vi "Save Excel Reports.vi"(11 "NI_report in":refnum<class "NI_report.lvclass">) -> ()   [LabVIEW 2019]
uses:
  <vilib>/Utility/NIReport.llb/NI_report.lvclass
  Global Tektronix Report Cells.vi
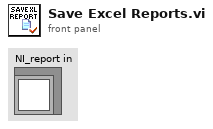
[diagram p1: front panel]
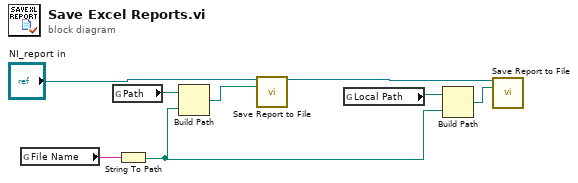
[diagram p0: block diagram]
diagram:
  n1 = global read "Global Tektronix Report Cells.vi" "File Name"() -> (w5:string)
  n2 = global read "Global Tektronix Report Cells.vi" "Path"() -> (w4:path)
  n3 = String To Path(string=w5) -> (path=w1:path)
  n4 = Build Path(base path=w4, name or relative path=w1) -> (appended path=w3:path)
  n5 = call-dynamic "Save Report to File.vi"("report in"="NI_report in", "report file path"=w3) -> ("report out"=w6:refnum<class "NI_report.lvclass">)  [unwired: 12 in, 1 out]
  n6 = global read "Global Tektronix Report Cells.vi" "Local Path"() -> (w7:path)
  n7 = Build Path(base path=w7, name or relative path=w1) -> (appended path=w8:path)
  n8 = call-dynamic "Save Report to File.vi"("report in"=w6, "report file path"=w8) -> ()  [unwired: 12 in, 2 out]
